vi "FABR-Read Data.vi"(0 "Data files":path[](array[path]), 7 "Threshold Estimation":T1={"Tmin (ms)"=1.0, "Tmax (ms)"=6.0, "CC criterion"=0.35, "adjR2 criterion"=0.0}, 11 "error in (no error)":errorcluster) -> (4 "Analysis":T2, 15 "error out":errorcluster)   [LabVIEW 2020]
uses:
  Typedefs/FABR-Analysis State.ctl
  Threshold Estimation VIs/ABR3-Threshold Estimation Parameters.ctl
  epl-vi-lib/Utility VIs/Array Manipulation VIs/Array-Dimensions (2D).vi
panel:
  out "Header":T3
  # "Freq X Level X Time"
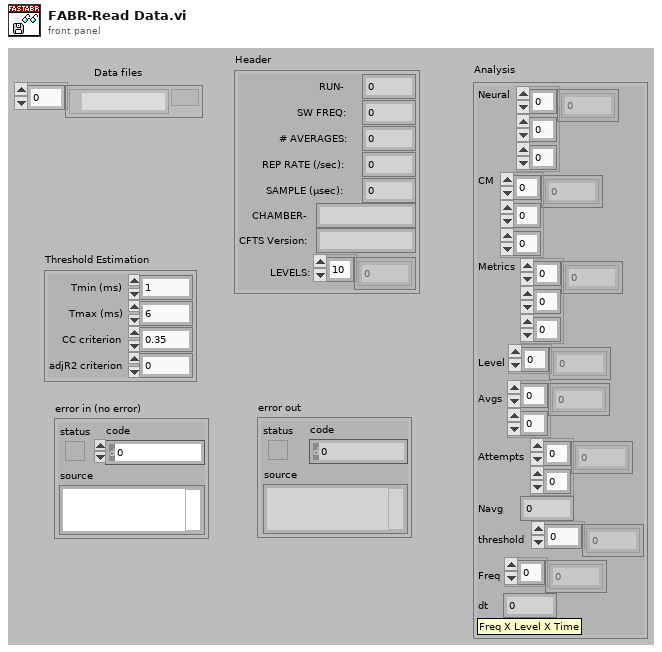
[diagram p1: front panel]
types:
  T1 = typedef "ABR3-Threshold Estimation Parameters.ctl" = cluster{"Tmin (ms)":dbl, "Tmax (ms)":dbl, "CC criterion":dbl, "adjR2 criterion":dbl}
  T2 = typedef "FABR-Analysis State.ctl" = cluster{"Neural":dbl[][][], "CM":dbl[][][], "Metrics":dbl[][][], "Level":dbl[], "Avgs":i32[][], "Attempts":i32[][], "Navg":i32, "threshold":dbl[], "Freq":dbl[], "dt":dbl}
  T3 = cluster{"RUN-":i32, "SW FREQ:":dbl, "# AVERAGES:":i32, "REP RATE (/sec):":dbl, "SAMPLE (µsec):":dbl, "CHAMBER-":string, "CFTS Version: ":string, "LEVELS:":dbl[]}
  T4 = typedef "ABR-Data Header.ctl" = cluster{"RUN-":i32, "SW FREQ:":dbl, "# AVERAGES:":i32, "REP RATE (/sec):":dbl, "SAMPLE (µsec):":dbl, "CHAMBER-":string, "CFTS Version: ":string, "LEVELS:":dbl[], "Date":timestamp, "Threshold:":dbl}
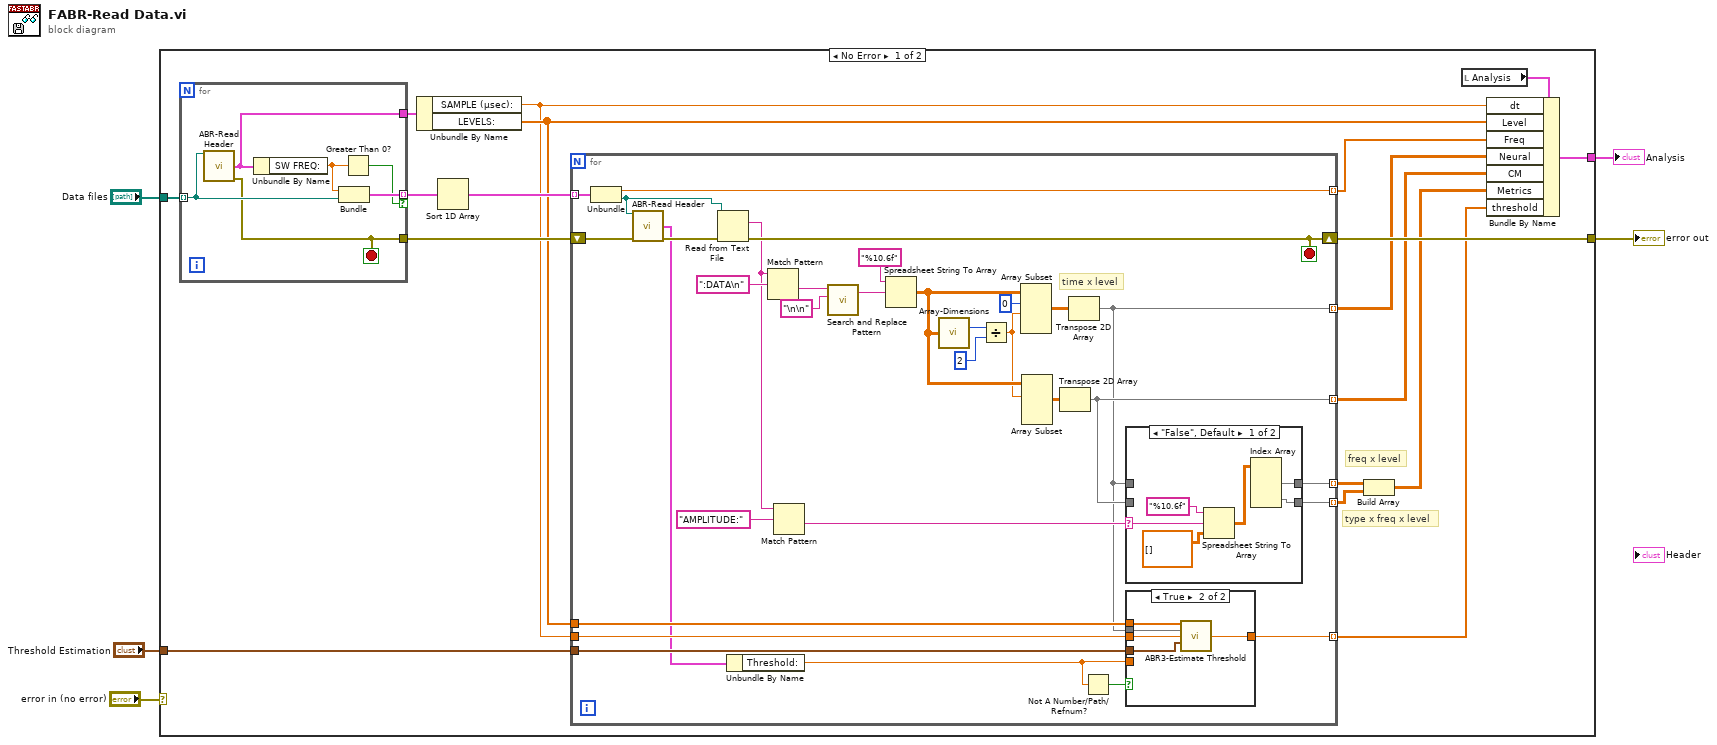
[diagram p0: block diagram]
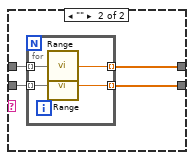
[diagram p3: hidden frame]
diagram:
  n1 = case shown="No Error" "error in (no error)" {
    selector: "error in (no error)" -> [_ w82]
    tunnel: [w15 w82] -> w4
    tunnel: "Data files" -> [w22 _]
    tunnel: [w23 _] -> w2
    tunnel: "Threshold Estimation" -> [w7 _]
    frame No Error {
      # "type x freq x level"
      # "freq x level"
      n2 = for {
        tunnel: w22 -> [w81] mode=indexing
        tunnel: [w80] -> w21 mode=indexing if=w78
        tunnel: [w77] -> w18
        tunnel: [w76] -> w16
        stop <- w76 stop-if-true
        n3 = call "ABR-Read Header.vi"("Path"=w81) -> ("Header"=w77:T4, "error out"=w76:errorcluster)  [unwired: 12 in, 1 out]
        n4 = Unbundle By Name(w77) -> ("SW FREQ:"=w79:dbl)
        n5 = Bundle("SW FREQ:"=w79, "Path"=w81) -> (w80:cluster{"SW FREQ:":dbl, "Path":path})  [unwired: 1 in]
        n6 = Greater Than 0?(x=w79) -> (x > 0?=w78:bool)
      }
      n7 = Unbundle By Name(w18) -> ("SAMPLE (µsec):"=w8:dbl, "LEVELS:"=w9:dbl[])
      n8 = Sort 1D Array(array=w21) -> (sorted array=w20:cluster{"SW FREQ:":dbl, "Path":path}[])
      n9 = for {
        tunnel: w20 -> [w55] mode=indexing
        tunnel: [w54] -> w17 mode=indexing
        shift-right: [w49] -> w15
        shift-left: w16 -> [w28]
        tunnel: [w33] -> w14 mode=indexing
        tunnel: [w43] -> w12 mode=indexing
        tunnel: [w39] -> w13 mode=indexing
        tunnel: [w38] -> w11 mode=indexing
        tunnel: w9 -> [w34]
        tunnel: w8 -> [w32]
        tunnel: w7 -> [w31]
        tunnel: [w30] -> w6 mode=indexing
        stop <- w49 stop-if-true
        # "time x level"
        n10 = Unbundle(w55) -> ("SW FREQ:"=w54:dbl, "Path"=w26:path)
        n11 = call "ABR-Read Header.vi"("Path"=w26, "error in"=w28) -> ("Header"=w25:T4, "error out"=w27:errorcluster)  [unwired: 11 in, 1 out]
        n12 = Read from Text File(file (use dialog)=w26, error in=w27) -> (text=w46:string, error out=w49:errorcluster)  [unwired: 2 in, 2 out]
        n13 = Unbundle By Name(w25) -> ("Threshold:"=w24:dbl)
        n14 = Match Pattern(string=w46, regular expression=":DATA\n" ("search string/char (-)")) -> (after substring=w37:string)  [unwired: 1 in, 3 out]
        n15 = Match Pattern(string=w46, regular expression="AMPLITUDE:") -> (after substring=w44:string)  [unwired: 1 in, 3 out]
        n16 = call <vilib>:"Search and Replace Pattern.vi"("string"=w37, "regular expression (\"\")"="\n\n" ("regular expression (\"\")")) -> ("result string"=w35:string)  [unwired: 3 in, 1 out]
        n17 = Spreadsheet String To Array(format string="%10.6f" ("spreadsheet string"), spreadsheet string=w35) -> (array=w41:dbl[][])  [unwired: 2 in]
        n18 = call-poly "Array-Dimensions.vi"("2D Array"=w41) -> ("# rows"=w51:i32)  [unwired: 13 in, 1 out]
        n19 = Divide(x=w51, y=2) -> (x/y=w40:dbl)
        n20 = Array Subset(array=w41, index (row)=0 ("index"), length (row)=w40) -> (w48:dbl[][])  [unwired: 2 in]
        n21 = Array Subset(array=w41, index (row)=w40) -> (w42:dbl[][])  [unwired: 3 in]
        n22 = Transpose 2D Array(2D array=w42) -> (transposed array=w39:dbl[][])
        n23 = Transpose 2D Array(2D array=w48) -> (transposed array=w33:dbl[][])
        n24 = Not A Number/Path/Refnum?(number/path/refnum=w24) -> (NaN/Path/Refnum?=w29:bool)
        n25 = case shown="\"False\", Default" w44 {
          selector: w44 -> [w67 _]
          tunnel: w33 -> [_ w71]
          tunnel: [w63 w69] -> w43
          tunnel: w39 -> [_ w70]
          tunnel: [w62 w68] -> w38
          frame "False", Default {
            n26 = Spreadsheet String To Array(format string="%10.6f" ("spreadsheet string"), spreadsheet string=w67, array type (2D Dbl)=dbl[][] []) -> (array=w64:dbl[][])  [unwired: 1 in]
            n27 = Index Array(array=w64) -> (element #1=w63:dbl[], element #2=w62:dbl[])  [unwired: 4 in]
          }
          frame "" {
            n28 = for {
              tunnel: w71 -> [w75] mode=indexing
              tunnel: [w74] -> w69 mode=indexing
              tunnel: w70 -> [w73] mode=indexing
              tunnel: [w72] -> w68 mode=indexing
              n29 = call "Range.vi"("Array"=w75) -> ("Range"=w74:dbl)
              n30 = call "Range.vi"("Array"=w73) -> ("Range"=w72:dbl)
            }
          }
        }
        n31 = case shown="True" w29 {
          tunnel: w34 -> [_ w61]
          tunnel: w33 -> [_ w60]
          tunnel: w32 -> [_ w59]
          tunnel: w31 -> [_ w58]
          tunnel: [w56 w57] -> w30
          tunnel: w24 -> [w56 _]
          frame False {
          }
          frame True {
            n32 = call "ABR3-Estimate Threshold.vi"("Level (in)"=w61, "Neural"=w60, "dt (us)"=w59, "Threshold Estimation"=w58) -> ("Threshold"=w57:dbl)  [unwired: 9 in, 2 out]
          }
        }
      }
      n33 = Build Array(w12, w11) -> (w10:dbl[][][])
      n34 = local read "Analysis"() -> (w19:T2)
      n35 = Bundle By Name(cluster=w19, "dt"=w8, "Level"=w9, "Freq"=w17, "Neural"=w14, "CM"=w13, "Metrics"=w10, "threshold"=w6) -> (w23:T2)
    }
    frame Error {
    }
  }
  "error out" <- w4
  "Analysis" <- w2
